vi "Power_Supply Global.vi"() -> ()   [LabVIEW 2018, in "Power_Supply Virtual.lvclass"]
uses:
  Power_Supply Virtual.lvclass
panel:
  in  "Power_Supply_Refs":refnum<class "Power_Supply Virtual.lvclass">[](array[class])
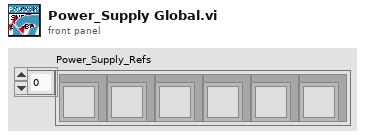
[diagram p1: front panel]
diagram:
